vi "K6221_GetSetPoint_Test.vi"() -> ()   [LabVIEW 2021]
panel:
  out "Control Value:Get All":cluster{"Name":string, "Variant Data":variant}[](array[cluster])
  in  "Data mac ip address":string="146.201.201.70"
  in  "port":u16=3375
  in  "error in (no error)":errorcluster
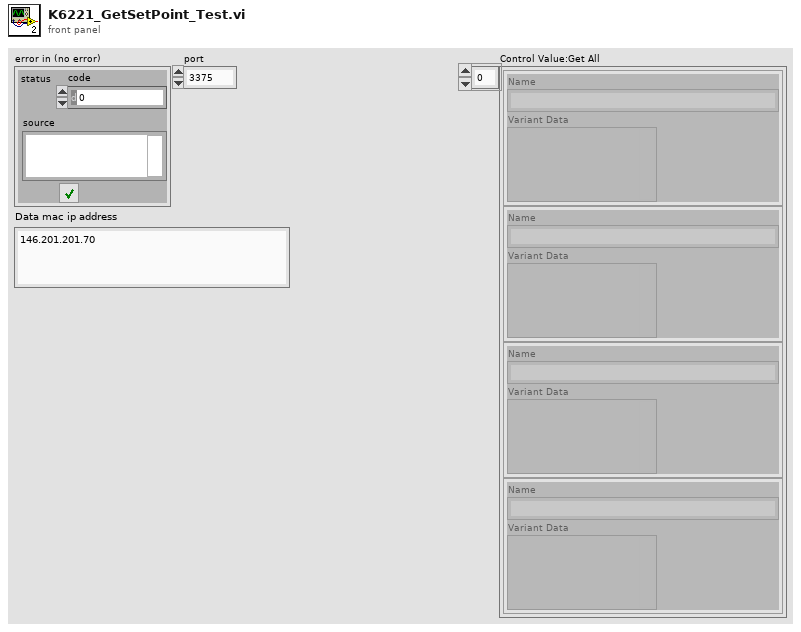
[diagram p1: front panel]
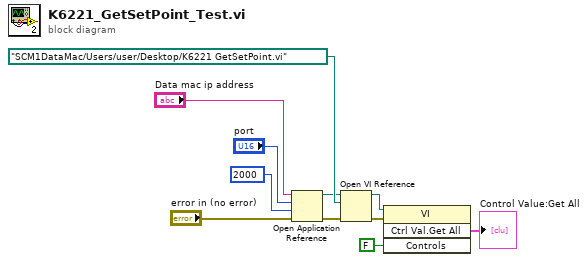
[diagram p0: block diagram]
diagram:
  n1 = Open Application Reference(8:"error in (no error)", 9:2000 ("timeout ms (60000)"), 10:"port", 11:"Data mac ip address") -> (0:w5:errorcluster, 3:w6:refnum<vi>)
  n2 = Open VI Reference(application reference (local)=w6, vi path=path "/SCM1DataMac/Users/user/Desktop/K6221 GetSetPoint.vi", error in (no error)=w5) -> (vi reference=w4:refnum<vi>, error out=w3:errorcluster)  [unwired: 3 in]
  n3 = invoke class="VI" method="Ctrl Val.Get All"(reference=w4, error in=w3, "Controls"=FALSE) -> ("Get All Control Values Variant"=→"Control Value:Get All":cluster{"Name":string, "Variant Data":variant}[])  [unwired: 1 in, 3 out]
